vi "SetTrig.vi"(8 "error in (no error)":errorcluster, 9 "TX trigger options":T1, 10 "Port":string(combo), 11 "reference in":refnum<class "sim_MmW.lvclass">) -> (0 "error out":errorcluster, 3 "reference out":refnum<class "sim_MmW.lvclass">)   [LabVIEW 2019, in "sim_MmW.lvclass"]
uses:
  sim_MmW.lvclass
  Low-level/TypeDefs/TX trigger config.ctl
  FPGA/SubVIs/Utility/FPGA driver trigger source.ctl
  FPGA/SubVIs/Utility/FPGA driver trigger destination.ctl
  FPGA/SubVIs/Utility/FPGA Utility.lvlib
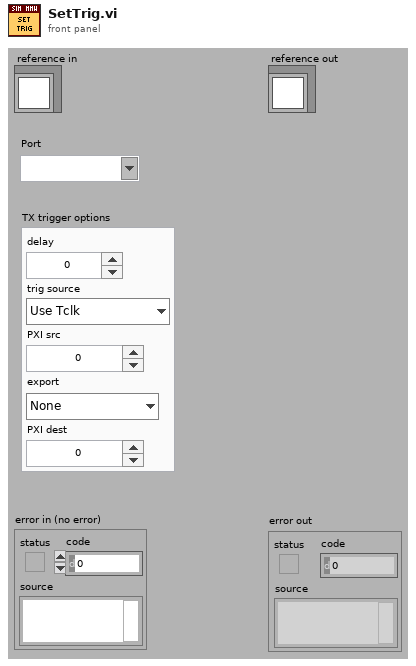
[diagram p1: front panel]
types:
  T1 = typedef "TX trigger config.ctl" = cluster{"delay":dbl, "trig source":T2, "PXI src":i32, "export":T3, "PXI dest":i32}
  T2 = typedef "FPGA Utility.lvlib/FPGA driver trigger source.ctl" = enum16{"Use Tclk", "PXI_Trig", "Aurora RX trig"}
  T3 = typedef "FPGA Utility.lvlib/FPGA driver trigger destination.ctl" = enum16{"None", "Source trig", "Synced trig", "Delayed sync"}
  T4 = typedef "sim_MmW.lvclass/ObjectAttributesRef.ctl" = refnum<data-value>
  T5 = typedef "sim_MmW.lvclass/ObjectAttributes.ctl" = cluster{"RF config":T6, "RX samples":i32, "Downloaded Bursts":map{string, refnum<class "mmWave data.lvclass">}, "TX Fs":dbl, "RX Fs":dbl, "burst sequence":string[], "Burst mode":T7}
  T6 = typedef "mmWave HW Control.lvlib/HW TXRX RF config cluster.ctl" = cluster{"TX.Frequency":dbl, "TX.Gain":dbl, "TX.mmWave adapter":string, "RX.Frequency":dbl, "RX.Gain":dbl, "RX.mmWave adapter":string}
  T7 = typedef "mmWave instrument.lvclass/BurstMode.ctl" = enum16{"burst", "continuous"}
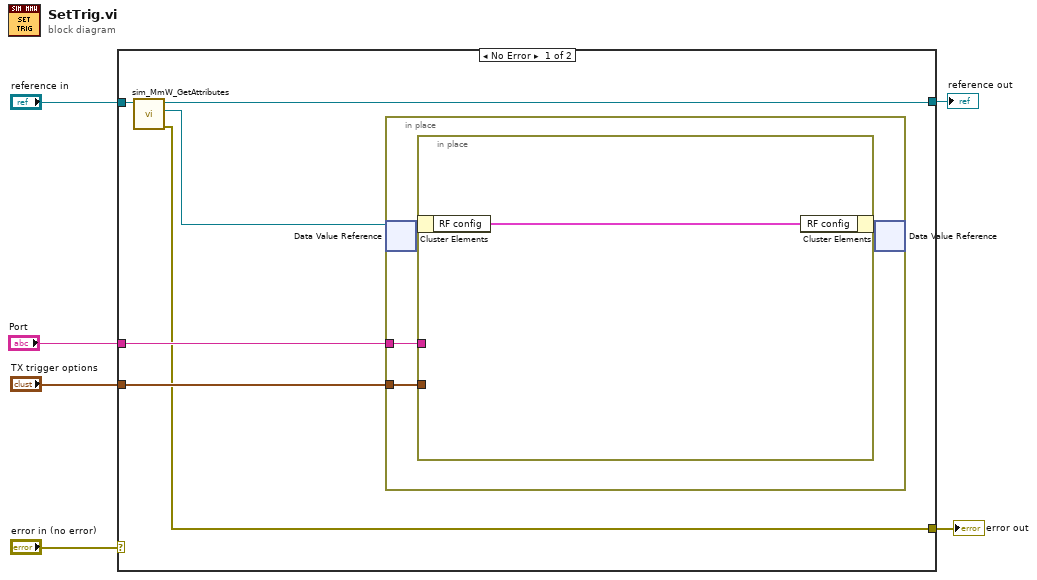
[diagram p0: block diagram]
diagram:
  n1 = case shown="No Error" "error in (no error)" {
    selector: "error in (no error)" -> [_ w19]
    tunnel: [w7 w19] -> w5
    tunnel: [w12 w18] -> w3
    tunnel: "reference in" -> [w11 w18]
    tunnel: "Port" -> [w9 _]
    tunnel: "TX trigger options" -> [w8 _]
    frame No Error {
      n2 = call "sim_MmW_GetAttributes.vi"("reference in"=w11) -> ("error out"=w7:errorcluster, "attributes ref"=w10:T4, "reference out"=w12:refnum<class "sim_MmW.lvclass">)  [unwired: 7 in, 1 out]
      n3 = in-place {
        in-place-border: w9 -> [w14]
        in-place-border: w8 -> [w13]
        n4 = in-place-dvr #1(w10) -> (w16:T5)  [unwired: 1 out]
        n5 = in-place {
          in-place-border: w14 -> [_]
          in-place-border: w13 -> [_]
          n6 = in-place-cluster #2(w16) -> ("RF config"=w17:T6)
          n7 = in-place-cluster #2("RF config"=w17) -> (w15:T5)
        }
        n8 = in-place-dvr #1(w15) -> ()  [unwired: 2 out]
      }
    }
    frame Error {
    }
  }
  "error out" <- w5
  "reference out" <- w3
